vi "MultiD Array to 1D Array of VArrays.vi"(8 "error in (no error)":errorcluster, 10 "MultiD Array":variant) -> (0 "error out":errorcluster, 2 "Array of VArrays":variant[](array[variant]))   [LabVIEW 2019, in "JKI JSON Serialization.lvlib" / "JSON Serializer.lvclass"]
doc: "JKI JSON 1.1.10.37\nTomi Maila - JKI\nCopyright (c) 2017, JKI"
uses:
  JSON Serializer.lvclass
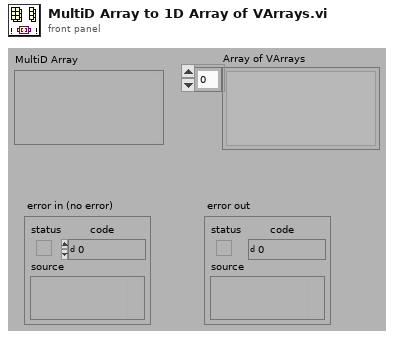
[diagram p1: front panel]
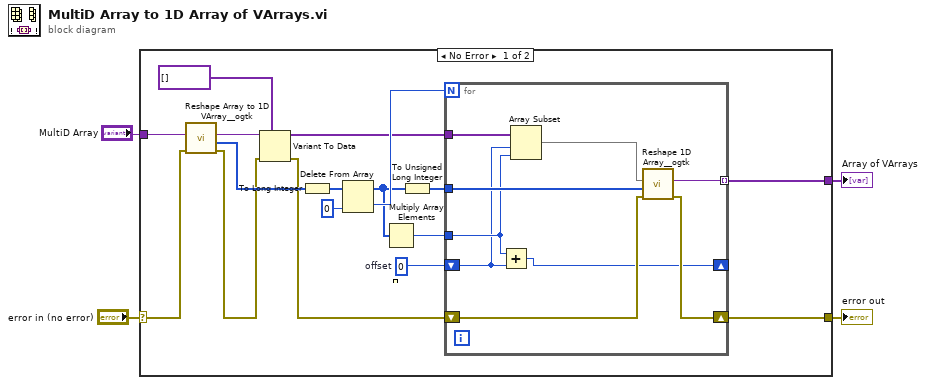
[diagram p0: block diagram]
diagram:
  n1 = case shown="No Error" "error in (no error)" {
    selector: "error in (no error)" -> [w20 w31]
    tunnel: [w13 w31] -> w4
    tunnel: [w7 _] -> w1
    tunnel: "MultiD Array" -> [w21 _]
    frame No Error {
      w16 = 0  # offset
      n2 = call "Reshape Array to 1D VArray__ogtk.vi"("error in (no error)"=w20, "MultiD Array"=w21) -> ("error out"=w10:errorcluster, "Size(s)"=w19:u32[], "1D VArray"=w12:variant)  [unwired: 7 in]
      n3 = Variant To Data(error in=w10, type=variant[] [], Variant=w12) -> (data=w11:variant[], error out=w9:errorcluster)
      n4 = To Long Integer(number=w19) -> (32bit integer=w6:i32[])
      n5 = Delete From Array(array=w6, index=0) -> (deleted portion=w17:i32, array with subset deleted=w15:i32[])  [unwired: 1 in]
      n6 = Multiply Array Elements(1:w15) -> (0:w14:i32)
      n7 = To Unsigned Long Integer(number=w15) -> (unsigned 32bit integer=w5:u32[])
      n8 = for {
        N: w17 -> [_]
        tunnel: w5 -> [w30]
        tunnel: w11 -> [w26]
        shift-right: [w28] -> w13
        shift-left: w9 -> [w29]
        shift-right: [w27] -> _
        shift-left: w16 -> [w23]
        tunnel: w14 -> [w24]
        tunnel: [w22] -> w7 mode=indexing
        n9 = Add(x=w24, y=w23) -> (x+y=w27:i32)
        n10 = Array Subset(array=w26, index=w23, length=w24) -> (w25:variant[])
        n11 = call "Reshape 1D Array__ogtk.vi"("error in (no error)"=w29, "Size(s)"=w30, "1D Array"=w25) -> ("error out"=w28:errorcluster, "Reshaped VArray"=w22:variant)  [unwired: 7 in]
      }
    }
    frame Error {
    }
  }
  "error out" <- w4
  "Array of VArrays" <- w1
